vi "hse-configuration_WriteIntegerKey.vi"(6 "Value":i32, 8 "error in (no error)":errorcluster, 9 "Key":string, 10 "Section":string, 11 "hse-config-ini in":refnum<class "hse-config-ini.lvclass">) -> (0 "error out":errorcluster, 3 "hse-config-ini out":refnum<class "hse-config-ini.lvclass">)   [LabVIEW 2020, in "hse-config-ini.lvclass"]
doc: "Writes the string configuration <b>value</b> identified by <b>section</b> and <b>key</b> to the configuration object and the config source\n\n____\nHAMPEL SOFTWARE ENGINEERING v3.8.0 (2023-12-18 14:41)"
uses:
  hse-config-ini.lvclass
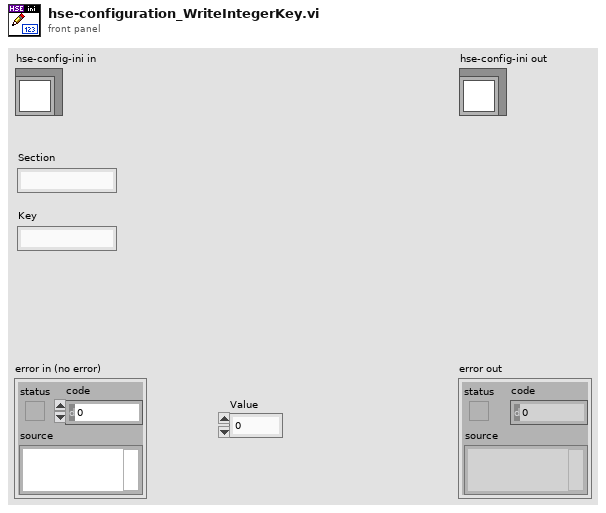
[diagram p1: front panel]
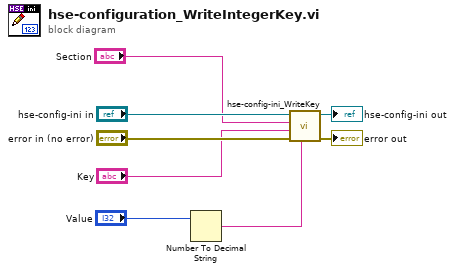
[diagram p0: block diagram]
diagram:
  n1 = Number To Decimal String(number="Value") -> (decimal integer string=w1:string)  [unwired: 1 in]
  n2 = call "hse-config-ini_WriteKey.vi"("Value"=w1, "error in (no error)"="error in (no error)", "Key"="Key", "Section"="Section", "hse-config-ini in"="hse-config-ini in") -> ("error out"=→"error out":errorcluster, "hse-config-ini out"=→"hse-config-ini out":refnum<class "hse-config-ini.lvclass">)  [unwired: 5 in]
